vi "conjugate_gradient(SubVI).vi"(4 "Tolerancja":dbl, 8 "Initial Guess":dbl[](array[numeric]), 10 "b":dbl[](array[numeric]), 11 "A":dbl[][](array[numeric])) -> (2 "Wykonana iczba Iteracji":i32, 3 "Gradientów Sprzê¿onych":dbl[](array[numeric]))   [LabVIEW 2020]
uses:
  <vilib>/addons/Multicore Analysis and Sparse Matrix/BLAS/_blas/dgemv - General Matrix-Vector Product (DBL).vi
  <vilib>/Analysis/Matrix/Numeric/Conversions/Array To Matrix - RA.vi
  <vilib>/Analysis/Matrix/NI_Matrix.lvlib
  <vilib>/addons/Multicore Analysis and Sparse Matrix/BLAS/NI_MASM_BLAS.lvlib
panel:
  out "Wczesny stop":bool
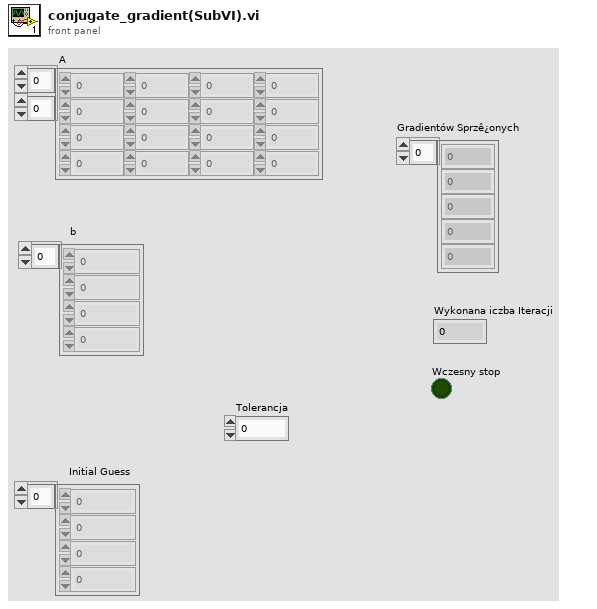
[diagram p1: front panel]
types:
  T1 = typedef "NI_Matrix.lvlib/RealMatrix.ctl" = dbl[][]
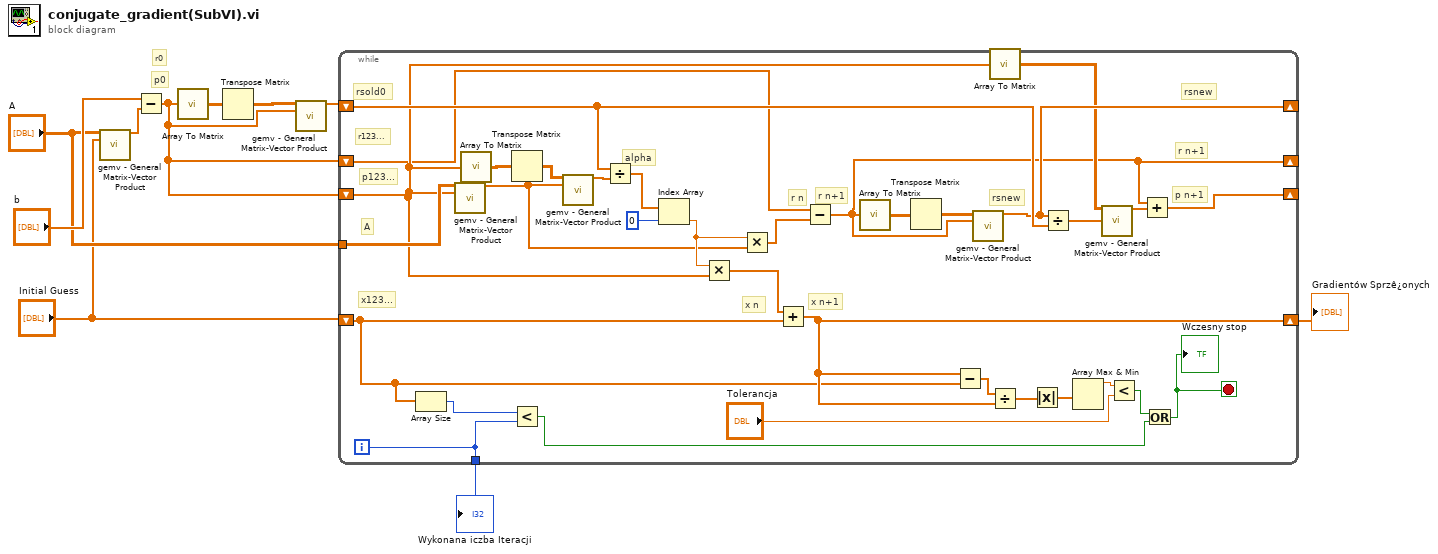
[diagram p0: block diagram]
diagram:
  # "p0"
  # "r0"
  n1 = call-poly <vilib>:"gemv - General Matrix-Vector Product.vi"("A"="A", "x"="Initial Guess") -> ("dgemv"=w10:dbl[])  [unwired: 12 in, 1 out]
  n2 = Subtract(x="b", y=w10) -> (x-y=w5:dbl[])
  n3 = call-poly <vilib>:"Array To Matrix.vi"("Real 1D Array"=w5) -> ("Real Matrix (Column Vector)"=w8:T1)
  n4 = Transpose Matrix(1:w8) -> (0:w7:T1)
  n5 = call-poly <vilib>:"gemv - General Matrix-Vector Product.vi"("A"=w7, "x"=w5) -> ("dgemv"=w6:dbl[])  [unwired: 12 in, 1 out]
  n6 = while {
    tunnel: "A" -> [w39]
    shift-right: [w18] -> w4
    shift-left: "Initial Guess" -> [w17]
    shift-right: [w24] -> _
    shift-left: w5 -> [w26]
    shift-right: [w22] -> _
    shift-left: w6 -> [w28]
    shift-right: [w20] -> _
    shift-left: w5 -> [w23]
    tunnel: [w15] -> w3
    i -> [w15]
    stop <- w12 stop-if-true
    # "rsold0"
    # "r n+1"
    # "rsnew"
    # "p n+1"
    # "rsnew"
    # "r n+1"
    # "r n"
    # "x n"
    # "x n+1"
    # "x123..."
    # "alpha"
    # "A"
    # "p123..."
    # "r123..."
    n7 = Array Size(array=w17) -> (size(s)=w16:i32)
    n8 = call-poly <vilib>:"gemv - General Matrix-Vector Product.vi"("A"=w39, "x"=w26) -> ("dgemv"=w31:dbl[])  [unwired: 12 in, 1 out]
    n9 = call-poly <vilib>:"Array To Matrix.vi"("Real 1D Array"=w26) -> ("Real Matrix (Column Vector)"=w38:T1)
    n10 = Transpose Matrix(1:w38) -> (0:w19:T1)
    n11 = Less?(x=w16, y=w15) -> (x < y?=w14:bool)
    n12 = call-poly <vilib>:"gemv - General Matrix-Vector Product.vi"("A"=w19, "x"=w31) -> ("dgemv"=w11:dbl[])  [unwired: 12 in, 1 out]
    n13 = Divide(x=w28, y=w11) -> (x/y=w37:dbl[])
    n14 = Index Array(array=w37, index=0) -> (element=w33:dbl)
    n15 = Multiply(x=w33, y=w26) -> (x*y=w34:dbl[])
    n16 = Multiply(x=w33, y=w31) -> (x*y=w32:dbl[])
    n17 = Add(x=w34, y=w17) -> (x+y=w18:dbl[])
    n18 = Subtract(x=w23, y=w32) -> (x-y=w20:dbl[])
    n19 = call-poly <vilib>:"Array To Matrix.vi"("Real 1D Array"=w20) -> ("Real Matrix (Column Vector)"=w30:T1)
    n20 = Transpose Matrix(1:w30) -> (0:w29:T1)
    n21 = Subtract ("Subtract.vi")(x=w18, y=w17) -> (x-y=w43:dbl[])
    n22 = call-poly <vilib>:"gemv - General Matrix-Vector Product.vi"("A"=w29, "x"=w20) -> ("dgemv"=w22:dbl[])  [unwired: 12 in, 1 out]
    n23 = call-poly <vilib>:"Array To Matrix.vi"("Real 1D Array"=w26) -> ("Real Matrix (Column Vector)"=w21:T1)
    n24 = Divide(x=w43, y=w18) -> (x/y=w42:dbl[])
    n25 = Absolute Value ("Absolute Value.vi")(x=w42) -> (abs(x)=w35:dbl[])
    n26 = Divide(x=w22, y=w28) -> (x/y=w27:dbl[])
    n27 = Array Max & Min(array=w35) -> (max value=w41:dbl)  [unwired: 3 out]
    n28 = call-poly <vilib>:"gemv - General Matrix-Vector Product.vi"("A"=w21, "x"=w27) -> ("dgemv"=w25:dbl[])  [unwired: 12 in, 1 out]
    n29 = Less?(x=w41, y="Tolerancja") -> (x < y?=w13:bool)
    n30 = Add(x=w20, y=w25) -> (x+y=w24:dbl[])
    n31 = Or(x=w13, y=w14) -> (x .or. y?=w12:bool)
    "Wczesny stop" <- w12
  }
  "Gradientów Sprzê¿onych" <- w4
  "Wykonana iczba Iteracji" <- w3
